vi "Tag.lookup_lua.vi"(5 "LuaVIEW reference":T1) -> (15 "error out":errorcluster)   [LabVIEW 2012]
doc: "Looks up the number tag with the provided name in the collection of live tags and returns a new tag object that allows that tag to be operated upon. This function is typically called in the initialisation section of a script for all required tags so as to ensure that the script fails at an early stage when not all these tags exist.\n\nThe returned tag object has an I32:read_index attribute that, after this function returns, is set to the write index, that is, it specifies the position of the next point to be written to the tag. The read_index is used to determine what point to read when calling the <code>read</code> method. Use the <code>seek</code> or <code>index</code> methods to change read_index. Note that each call to this function returns a new tag object with its own private read_index. This allows there to be multiple independent readers of tag.\n\nThe read_index overflows to -2^31 at +2^31. The buffering and reading is designed to continue without a hitch when this occurs, but it means that the read_index <b>cannot</b> be interpreted as an absolute value. It only makes sense as a value relative to another buffer index, with differences calculable via signed 32 bit integer arithmetic only.\n\nIn addition, the returned tag object has a str:unit attribute that specifies the physical unit of the tag, or is an empty string when the tag is dimensionless. The optional second argument causes verification that the unit of the tag is as the script expects. It is advisable to specify it when your script makes assumptions as to the unit of the tag.\n\nSince tag names are guaranteed to be valid Lua identifiers, it is possible to assign the returned object to a variable with the same name as the tag. This is <b>not</b> advisable when the tag might change, or it is likely that a copy of the script will be made to serve a different set of tags, since then the script would have to be changed in multiple places (to keep the tag name and various uses of the object variable mutually consistent) instead of just a single place. In such cases it is better to use a short generic variable name, or a name that reflects the role of the tag in the context of the script's actions.\nParameters:\nstr:name, name of the tag for which to return an object.\n[str:unit], expected unit.\nResults:\nobj:tag, LuaVIEW object referencing the specified number tag.\nErrors:\nNo live tag with the provided name exists.\nActual unit does not match expected unit.\nSpecified tag is not a number tag.\nData logger not initialized."
uses:
  luaview/typedefs/t_LuaVIEW Reference.ctl
  typedefs/t_DataLog Tag Hash Methods.ctl
  typedefs/t_DataLog Tag Info List Methods.ctl
  typedefs/t_DataLog Tag Buffers Methods.ctl
  luaview/subvis/private/LuaVIEW Pull (string).vi
  luaview/subvis/private/LuaVIEW Push (object).vi
  luaview/subvis/private/LuaVIEW Push (I32).vi
  luaview/subvis/private/LuaVIEW Push (string).vi
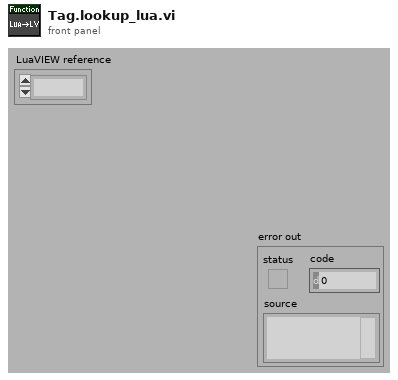
[diagram p1: front panel]
types:
  T1 = typedef "t_LuaVIEW Reference.ctl" = refnum<k1>
  T2 = typedef "t_DataLog Tag Info List Methods.ctl" = enum16{"initialize", "create", "create empty", "rename", "delete", "test tag", "get", "get by name", "get default", "get list", "get path", "get subsets", "set subsets", "set config", "set capacity", "#tags", "go live", "set unlocked", "set mirrored"}
  T3 = typedef "t_DataLog Tag Hash Methods.ctl" = enum16{"initialize", "add tag", "index tag", "lookup", "#tags", "cleanup", "write recovery", "read recovery", "delete recovery"}
  T4 = typedef "t_DataLog Tag Config.ctl" = cluster{"name":string, "unit":string, "temporal":T5, "value":T6, "index":i32, "capacity":i32, "is meta?":bool, "mincapacity":i32, "deadband":dbl, "limit delay":dbl, "format":T7, "precision":u8, "undefine":bool, "update":bool, "update period":u16, "expression":string, "description":string, "logging algorithm":T8, "logging parameters":dbl[]}
  T5 = typedef "t_DataLog Temporal Types.ctl" = enum16{"set&hold", "sample", "event"}
  T6 = typedef "t_DataLog Value Types.ctl" = enum16{"number", "string"}
  T7 = typedef "t_DataLog Numerical Format.ctl" = enum8{"fractional", "exponential", "engineering"}
  T8 = typedef "t_DataLog Logging Algorithms.ctl" = enum16{"nothing", "changes", "everything", "every Nth", "time threshold", "value threshold + prior", "t or v threshold", "t or v threshold + prior"}
  T9 = typedef "t_DataLog Tag Buffers Methods.ctl" = enum16{"initialize", "inert", "write", "read", "read oldest", "read last", "cleanup"}
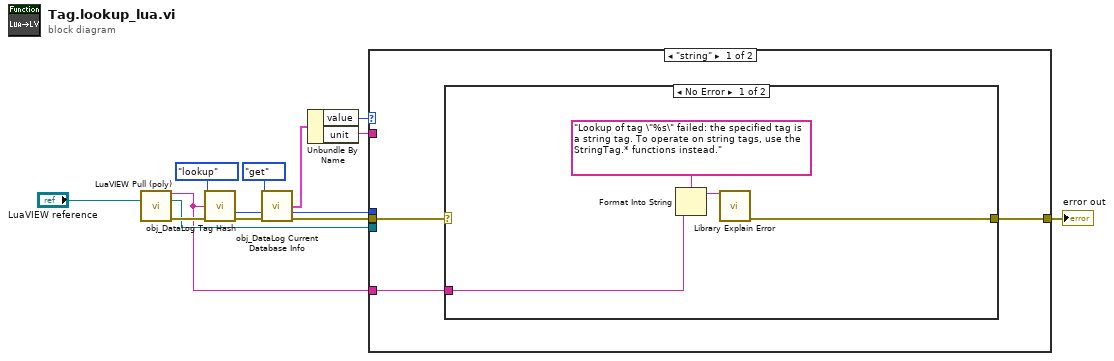
[diagram p0: block diagram]
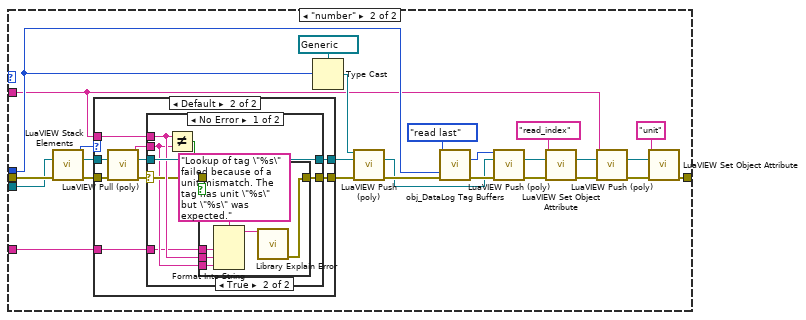
[diagram p3: hidden frame]
diagram:
  n1 = call-poly "LuaVIEW Pull (poly).vi"("LuaVIEW reference in"="LuaVIEW reference") -> ("string"=w2:string, "LuaVIEW reference out"=w4:T1, "error out"=w12:errorcluster)  [unwired: 12 in]
  n2 = call "obj_DataLog Tag Hash.vi"("method"=t_DataLog_Tag_Hash_Methods."lookup", "tag in"=w2, "error in (no error)"=w12) -> ("tag index out"=w9:i32, "error out"=w10:errorcluster)  [unwired: 9 in, 2 out]
  n3 = call "obj_DataLog Current Database Info.vi"("method"=t_DataLog_Tag_Info_List_Methods."get", "tag index/change#"=w9, "error in (no error)"=w10) -> ("tag config out"=w6:T4, "dup tag index"=w8:i32, "error out"=w5:errorcluster)  [unwired: 6 in, 4 out]
  n4 = Unbundle By Name(w6) -> ("value"=w1:T6, "unit"=w3:string)
  n5 = case shown="\"string\"" w1 {
    tunnel: [w17 w33] -> w11
    tunnel: w8 -> [_ w32]
    tunnel: w5 -> [w16 w29]
    tunnel: w4 -> [_ w28]
    tunnel: w3 -> [_ w25]
    tunnel: w2 -> [w15 w24]
    frame "string" {
      n6 = case shown="No Error" w16 {
        selector: w16 -> [_ w22]
        tunnel: [w18 w22] -> w17
        tunnel: w15 -> [w19 _]
        frame No Error {
          n7 = Format Into String(format string="Lookup of tag \"%s\" failed: the specified tag is a string tag. To operate on string tags, use the StringTag.* functions instead." ("string"), w19) -> (resulting string=w21:string)  [unwired: 2 in, 1 out]
          n8 = call "Library Explain Error.vi"("explanation prefix (none)"=w21) -> ("explained error"=w18:errorcluster)  [unwired: 14 in]
        }
        frame Error {
        }
      }
    }
    frame "number" {
      n9 = call "LuaVIEW Stack Elements.vi"("LuaVIEW reference in"=w28, "error in (no error)"=w29) -> ("elements"=w26:i32, "LuaVIEW reference out"=w27:T1, "error out"=w30:errorcluster)  [unwired: 11 in]
      n10 = case shown="Default" w26 {
        tunnel: [w50 w53] -> w31
        tunnel: w30 -> [w49 w59]
        tunnel: w27 -> [w50 w58]
        tunnel: w25 -> [_ w57]
        tunnel: w24 -> [_ w51]
        tunnel: [w49 w52] -> w23
        frame 0 {
        }
        frame Default {
          n11 = call-poly "LuaVIEW Pull (poly).vi"("LuaVIEW reference in"=w58, "error in (no error)"=w59) -> ("string"=w56:string, "LuaVIEW reference out"=w54:T1, "error out"=w55:errorcluster)  [unwired: 11 in]
          n12 = case shown="No Error" w55 {
            selector: w55 -> [w63 w74]
            tunnel: w57 -> [w64 _]
            tunnel: w56 -> [w61 _]
            tunnel: w54 -> [w66 w75]
            tunnel: [w66 w75] -> w53
            tunnel: [w62 w74] -> w52
            tunnel: w51 -> [w60 _]
            frame No Error {
              n13 = Not Equal?(x=w64, y=w61) -> (x != y?=w65:bool)
              n14 = case shown="True" w65 {
                tunnel: w64 -> [_ w72]
                tunnel: w63 -> [w67 _]
                tunnel: [w67 w69] -> w62
                tunnel: w61 -> [_ w71]
                tunnel: w60 -> [_ w73]
                frame False {
                }
                frame True {
                  n15 = Format Into String(format string="Lookup of tag \"%s\" failed because of a unit mismatch. The tag has unit \"%s\" but \"%s\" was expected." ("string"), w73, w72, w71) -> (resulting string=w70:string)  [unwired: 2 in, 1 out]
                  n16 = call "Library Explain Error.vi"("explanation prefix (none)"=w70) -> ("explained error"=w69:errorcluster)  [unwired: 14 in]
                }
              }
            }
            frame Error {
            }
          }
        }
      }
      n17 = Type Cast(type=refnum<vi> refnum ("object refnum"), x=w32) -> (*(type *) &x=w47:refnum<vi>)
      n18 = call-poly "LuaVIEW Push (poly).vi"("object refnum"=w47, "LuaVIEW reference in"=w31, "error in (no error)"=w23) -> ("LuaVIEW reference out"=w39:T1, "error out"=w44:errorcluster)  [unwired: 11 in]
      n19 = call "obj_DataLog Tag Buffers.vi"("method"=t_DataLog_Tag_Buffers_Methods."read last", "tag index"=w32, "error in (no error)"=w44) -> ("read index out"=w42:i32, "error out"=w43:errorcluster)  [unwired: 8 in, 3 out]
      n20 = call-poly "LuaVIEW Push (poly).vi"("I32"=w42, "LuaVIEW reference in"=w39, "error in (no error)"=w43) -> ("LuaVIEW reference out"=w46:T1, "error out"=w45:errorcluster)  [unwired: 11 in]
      n21 = call "LuaVIEW Set Object Attribute.vi"("key"="read_index", "LuaVIEW reference in"=w46, "error in (no error)"=w45) -> ("LuaVIEW reference out"=w36:T1, "error out"=w37:errorcluster)  [unwired: 11 in]
      n22 = call-poly "LuaVIEW Push (poly).vi"("string"=w25, "LuaVIEW reference in"=w36, "error in (no error)"=w37) -> ("LuaVIEW reference out"=w35:T1, "error out"=w34:errorcluster)  [unwired: 11 in]
      n23 = call "LuaVIEW Set Object Attribute.vi"("key"="unit", "LuaVIEW reference in"=w35, "error in (no error)"=w34) -> ("error out"=w33:errorcluster)  [unwired: 11 in, 1 out]
    }
  }
  "error out" <- w11
